vi "SessionManagementService GetMultiplexerSessions.vi"(6 "contextId":T1, 8 "error in":errorcluster, 9 "timeout (ms)":i32=-1, 10 "Request Data":T5, 11 "gRPC ID":T1) -> (0 "error out":errorcluster, 2 "Response Data":T2, 3 "gRPC ID out":T1)   [LabVIEW 2020, in "MeasurementLink Session Management Client.lvlib"]
uses:
  MeasurementLink Session Management Client.lvlib
  <vilib>/gRPC/LabVIEW gRPC Library/Shared/grpcId.ctl
  RPC Messages/ni_measurementlink_sessionmanagement_v1_GetMultiplexerSessionsRequest.ctl
  RPC Messages/ni_measurementlink_PinMapContext.ctl
  RPC Messages/ni_measurementlink_sessionmanagement_v1_GetMultiplexerSessionsResponse.ctl
  RPC Messages/ni_measurementlink_sessionmanagement_v1_MultiplexerSessionInformation.ctl
  RPC Messages/nidevice_grpc_Session.ctl
  RPC Messages/ni_measurementlink_sessionmanagement_v1_GetMultiplexerSessionsResponse_Flat.ctl
  RPC Messages/ni_measurementlink_sessionmanagement_v1_MultiplexerSessionInformation_Flat.ctl
  RPC Messages/nidevice_grpc_Session_Flat.ctl
  14035477-4c25-4107-8ed5-d0c4ef420ce5.vi
  RPC Messages/RichToFlatni_measurementlink_PinMapContext.vi
  <vilib>/gRPC/LabVIEW gRPC Library/Shared/TranslateGrpcError.vi
  <vilib>/gRPC/LabVIEW gRPC Library/Shared/Wait On Occurence.vi
  RPC Messages/FlatToRichni_measurementlink_sessionmanagement_v1_MultiplexerSessionInformation.vi
  RPC Messages/FlatToRichnidevice_grpc_Session.vi
  <vilib>/gRPC/LabVIEW gRPC Library/Server API/Server/Get Server DLL Path.vi
  <vilib>/Utility/error.llb/Error Cluster From Error Code.vi
  <vilib>/Utility/error.llb/Simple Error Handler.vi
  <vilib>/gRPC/LabVIEW gRPC Library/grpc-lvsupport-release.lvlib
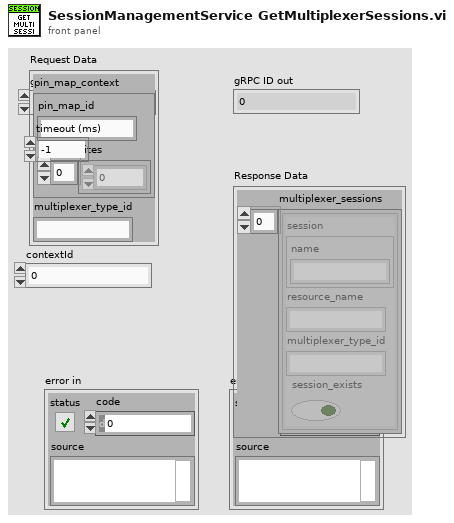
[diagram p1: front panel]
types:
  T1 = typedef "grpc-lvsupport-release.lvlib/grpcId.ctl" = u64
  T2 = typedef "MeasurementLink Session Management Client.lvlib/ni_measurementlink_sessionmanagement_v1_GetMultiplexerSessionsResponse.ctl" = cluster{"multiplexer_sessions":T3[]}
  T3 = typedef "MeasurementLink Session Management Client.lvlib/ni_measurementlink_sessionmanagement_v1_MultiplexerSessionInformation.ctl" = cluster{"session":T4, "resource_name":string, "multiplexer_type_id":string, "session_exists":bool}
  T4 = typedef "MeasurementLink Session Management Client.lvlib/nidevice_grpc_Session.ctl" = cluster{"name":string}
  T5 = typedef "MeasurementLink Session Management Client.lvlib/ni_measurementlink_sessionmanagement_v1_GetMultiplexerSessionsRequest.ctl" = cluster{"pin_map_context":T6, "multiplexer_type_id":string}
  T6 = typedef "MeasurementLink Session Management Client.lvlib/ni_measurementlink_PinMapContext.ctl" = cluster{"pin_map_id":string, "sites":i32[]}
  T7 = typedef "MeasurementLink Session Management Client.lvlib/ni_measurementlink_sessionmanagement_v1_GetMultiplexerSessionsResponse_Flat.ctl" = cluster{"multiplexer_sessions":T8[]}
  T8 = typedef "MeasurementLink Session Management Client.lvlib/ni_measurementlink_sessionmanagement_v1_MultiplexerSessionInformation_Flat.ctl" = cluster{"session":T9, "resource_name":string, "multiplexer_type_id":string, "session_exists":bool}
  T9 = typedef "MeasurementLink Session Management Client.lvlib/nidevice_grpc_Session_Flat.ctl" = cluster{"name":string}
  T10 = typedef "MeasurementLink Session Management Client.lvlib/ni_measurementlink_sessionmanagement_v1_GetMultiplexerSessionsRequest_Flat.ctl" = cluster{"pin_map_context":T11, "multiplexer_type_id":string}
  T11 = typedef "MeasurementLink Session Management Client.lvlib/ni_measurementlink_PinMapContext_Flat.ctl" = cluster{"pin_map_id":string, "sites":i32[]}
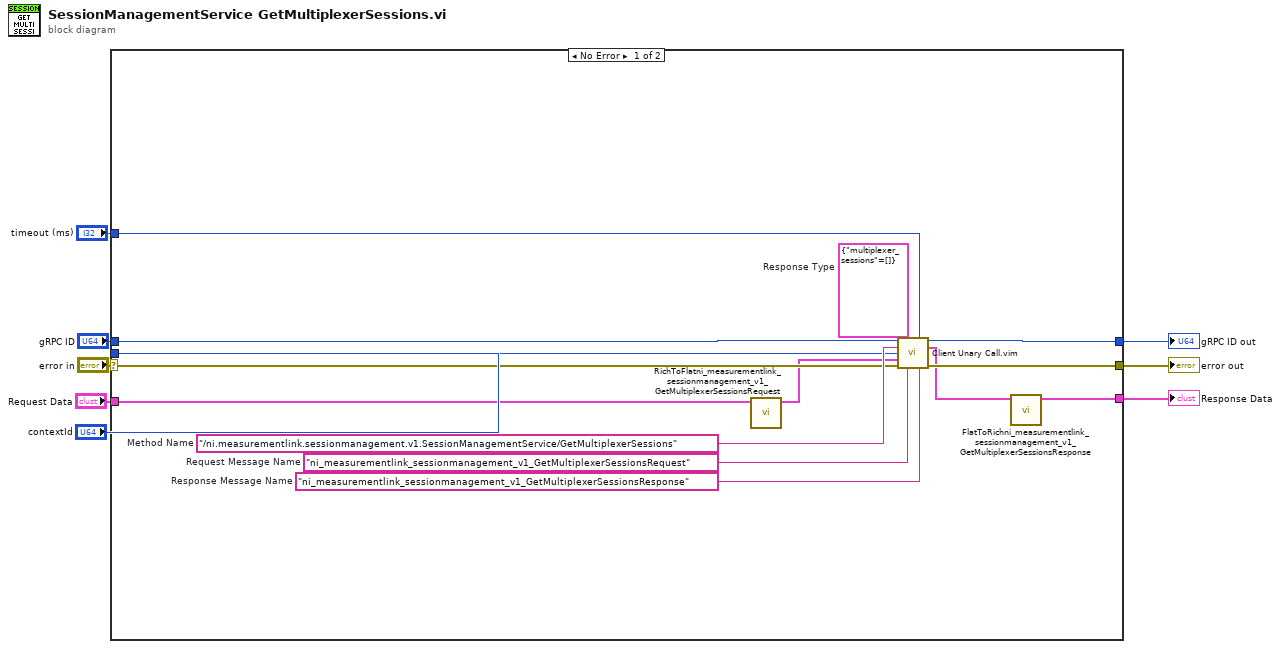
[diagram p0: block diagram]
diagram:
  n1 = case shown="No Error" "error in" {
    selector: "error in" -> [w18 w23]
    tunnel: [w17 w23] -> w7
    tunnel: "gRPC ID" -> [w16 w24]
    tunnel: [w15 w24] -> w5
    tunnel: "Request Data" -> [w12 _]
    tunnel: [w9 _] -> w3
    tunnel: "timeout (ms)" -> [w14 _]
    tunnel: "contextId" -> [w13 _]
    frame No Error {
      w19 = "ni_measurementlink_sessionmanagement_v1_GetMultiplexerSessionsResponse"  # Response Message Name
      w20 = "ni_measurementlink_sessionmanagement_v1_GetMultiplexerSessionsRequest"  # Request Message Name
      w21 = T7 {"multiplexer_sessions"=[]}  # Response Type
      w22 = "/ni.measurementlink.sessionmanagement.v1.SessionManagementService/GetMultiplexerSessions"  # Method Name
      n2 = call "RichToFlatni_measurementlink_sessionmanagement_v1_GetMultiplexerSessionsRequest.vi"("InputCluster"=w12) -> ("OutputCluster"=w11:T10)  [unwired: 10 in]
      n3 = call "Client Unary Call.vim"("ClientID in"=w16, "Response Type"=w21, "timeout (ms)"=w14, "Method Name"=w22, "contextId"=w13, "Request Data"=w11, "error in"=w18, "Request Message Name"=w20, "Response Message Name"=w19) -> ("ClientID out"=w15:u64, "Response Data"=w10:T7, "error out"=w17:errorcluster)  [unwired: 4 in]
      n4 = call "FlatToRichni_measurementlink_sessionmanagement_v1_GetMultiplexerSessionsResponse.vi"("InputCluster"=w10) -> ("OutputCluster"=w9:T2)  [unwired: 10 in]
    }
    frame Error {
    }
  }
  "error out" <- w7
  "gRPC ID out" <- w5
  "Response Data" <- w3
